vi "GetWorldCalibration.vi"(7 "error in":errorcluster) -> (27 "error out":errorcluster)   [LabVIEW 2015]
uses:
  <vilib>/vision/NI_Vision_Development_Module.lvlib
panel:
  out "Image Out":T1(plugin-control)
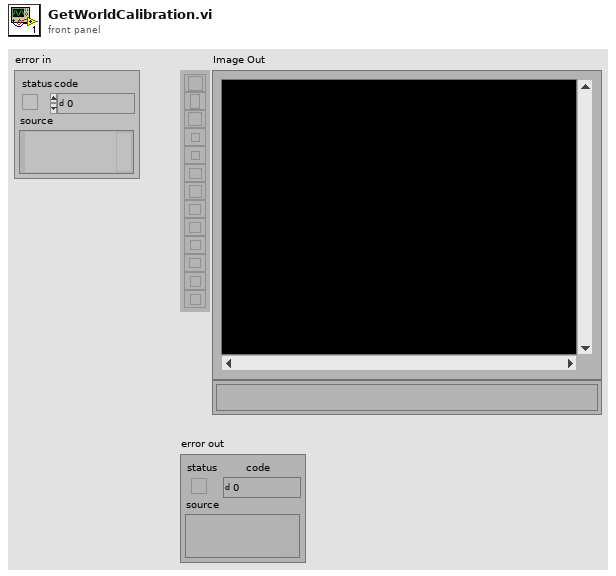
[diagram p1: front panel]
types:
  T1 = typedef "IMAQ Image.ctl" = refnum<image>
  T2 = enum32{"AutoM", "Close", "Dilate", "Erode", "Gradient", "Gradient out", "Gradient in", "Hit miss", "Open", "PClose", "POpen", "Thick", "Thin"}
  T3 = cluster{"Origin Pixel":cluster{"X":sgl, "Y":sgl}, "X Axis Pixel":cluster{"X":sgl, "Y":sgl}, "Axis Reference":u32}
  T4 = typedef "Image Type" = u32
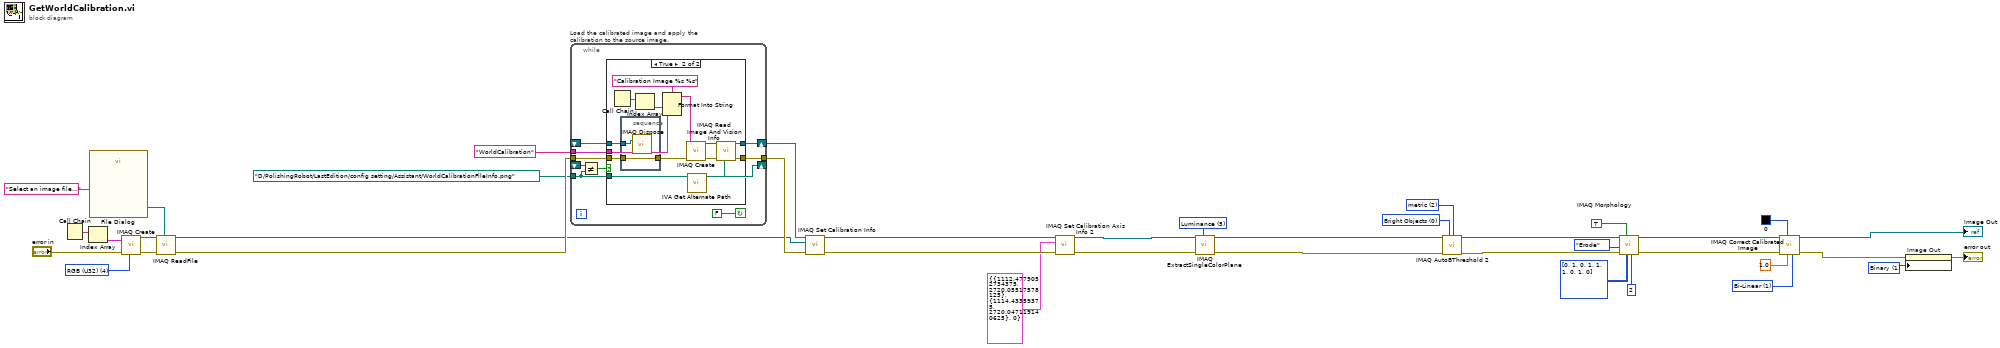
[diagram p0: block diagram]
diagram:
  w1 = u32 1 items=["Grayscale", "Binary", "Gradient", "Rainbow", "Temperature", "User Defined", "Binary 16 Bit", "Gradient 16 Bit", "Rainbow 16 Bit", "Temperature 16 Bit", "User Defined 16 Bit"] ("Palette Type")
  w8 = u32 1 items=["Zero Order", "Bi-Linear", "Quadratic", "Cubic Spline"] ("Interpolation Type")
  w15 = 2 items=["clustering", "entropy", "metric", "moments", "inter-class variance"] ("Method")
  w16 = u32 0 items=["Bright Objects", "Dark Objects"] ("Look For")
  w21 = 5 items=["Red", "Green", "Blue", "Hue", "Saturation", "Luminance", "Value", "Intensity"] ("Color Plane")
  w31 = T4 4 items=["Grayscale (U8)", "Grayscale (I16)", "Grayscale (SGL)", "Complex (CSG)", "RGB (U32)", "HSL (U32)", "RGB (U64)", "Grayscale (U16)"] ("Image Type")
  n1 = Call Chain() -> (call chain=w35:string[])
  n2 = Index Array(array=w35) -> (element=w34:string)  [unwired: 1 in]
  n3 = call "File Dialog"("prompt"="Select an image file...") -> ("selected path"=w32:path)  [unwired: 6 in, 8 out]
  n4 = call "IMAQ Create"("Image Name"=w34, "Image Type"=w31, "error in (no error)"="error in") -> ("New Image"=w38:T1, "error out"=w37:errorcluster)  [unwired: 1 in, 1 out]
  n5 = call "IMAQ ReadFile"("File Path"=w32, "error in (no error)"=w37, "Image"=w38) -> ("error out"=w39:errorcluster, "Image Out"=w26:T1)  [unwired: 2 in, 5 out]
  n6 = while "Load the calibrated image and apply the calibration to the source image." {
    shift-right: [w48] -> w29
    shift-left: _ -> [w47]
    tunnel: [w45] -> w28
    tunnel: w39 -> [w44]
    tunnel: path "D:/PolishingRobot/LastEdition/config setting/Assistant/WorldCalibrationFileInfo.png" ("File Path") -> [w40]
    tunnel: "WorldCalibration" ("Step Name") -> [w43]
    shift-right: [w40] -> _
    shift-left: _ -> [w42]
    stop <- FALSE continue-if-true
    n7 = Not Equal?(x=w42, y=w40) -> (x != y?=w41:bool)
    n8 = case shown="True" w41 {
      tunnel: [w50 w62] -> w48
      tunnel: w47 -> [w50 w54]
      tunnel: [w49 w59] -> w45
      tunnel: w44 -> [w49 w55]
      tunnel: w40 -> [_ w52]
      tunnel: w43 -> [_ w56]
      frame False {
      }
      frame True {
        n9 = Call Chain() -> (call chain=w58:string[])
        n10 = stacked-sequence {
          tunnel: w55 -> [w65]
          tunnel: w54 -> [w66]
          tunnel: [w65] -> w53
          frame #0 {
            n11 = call "IMAQ Dispose"("Image"=w66) -> ()  [unwired: 2 in, 4 out]
          }
        }
        n12 = Index Array(array=w58) -> (element=w57:string)  [unwired: 1 in]
        n13 = Format Into String(format string="Calibration Image %s %s" ("Image Name"), w57, w56) -> (resulting string=w64:string)  [unwired: 2 in, 1 out]
        n14 = call "IMAQ Create"("Image Name"=w64, "error in (no error)"=w53) -> ("New Image"=w61:T1, "error out"=w60:errorcluster)  [unwired: 2 in, 1 out]
        n15 = call <vilib>:"IVA Get Alternate Path.vi"("Path In"=w52) -> ("Path Out"=w51:path)  [unwired: 10 out]
        n16 = call "IMAQ Read Image And Vision Info"("File Path"=w51, "error in (no error)"=w60, "Image"=w61) -> ("error out"=w59:errorcluster, "Image Out"=w62:T1)  [unwired: 1 in, 6 out]
      }
    }
  }
  n17 = call "IMAQ Set Calibration Info"("error in (no error)"=w28, "Image Dst"=w26, "Image Src"=w29) -> ("error out"=w27:errorcluster, "Calibrated Image"=w23:T1)  [unwired: 1 in, 6 out]
  n18 = call-poly "IMAQ Set Calibration Axis Info 2"("error in (no error)"=w27, "Calibration Axis Info"=T3 {"Origin Pixel"={"X"=1112.4779, "Y"=2720.0552}, "X Axis Pixel"={"X"=1114.4336, "Y"=2720.047}, "Axis Reference"=0}, "Calibration Template Image In"=w23) -> ("error out"=w24:errorcluster, "Calibration Template Image Out"=w20:T1)  [unwired: 7 out]
  n19 = call "IMAQ ExtractSingleColorPlane"("Color Plane"=w21, "error in (no error)"=w24, "Image Src"=w20) -> ("error out"=w19:errorcluster, "Image Dst Out"=w18:T1)  [unwired: 1 in, 6 out]
  n20 = call "IMAQ AutoBThreshold 2"("Image Src"=w18, "Look For (Bright Objects)"=w16, "Method (clustering)"=w15, "error in (no error)"=w19) -> ("Image Dst Out"=w10:T1, "error out"=w17:errorcluster)  [unwired: 4 in, 6 out]
  n21 = call "IMAQ Morphology"("Number of iterations (1)"=2, "Structuring Element"=i32[][] [[0, 1, 0], [1, 1, 1], [0, 1, 0]], "Square/Hexa (Square)"=TRUE, "error in (no error)"=w17, "Operation"=T2."Erode", "Image Src"=w10) -> ("error out"=w9:errorcluster, "Image Dst Out"=w6:T1)  [unwired: 1 in, 3 out]
  n22 = call "IMAQ Correct Calibrated Image"("Interpolation Type"=w8, "Replace Value"=sgl 1.0, "Color Replace Value"=u32 0, "error in (no error)"=w9, "Image Src"=w6) -> ("error out"=w7:errorcluster, "Corrected Image"=→"Image Out":T1)  [unwired: 2 in, 3 out]
  n23 = property on="Image Out" class="ImageControl"(error in=w7, "Palette:Palette Type"=w1) -> (error out=→"error out":errorcluster)  [unwired: 1 in, 1 out]
